vi "Check Alarm-Error Consistency.vi"(8 "error in (no error)":errorcluster, 11 "STEP In":T1) -> (0 "error out":errorcluster, 2 "Array":bool[](array[boolean]), 3 "STEP out":T1)   [LabVIEW 2014, in "SeqLoop.lvlib"]
uses:
  TypeDefs/STEP.ctl
  TypeDefs/LogicParsedExpression.ctl
  Mimico Display/TypeDefs/Mimic Data.ctl
  Mimico Display/TypeDefs/BG Image.ctl
  Mimico Display/TypeDefs/mObject.ctl
  <vilib>/regexp/Match Regular Expression.xnode
  SeqLoop.lvlib
  Mimico Display/Mimico Display.lvlib
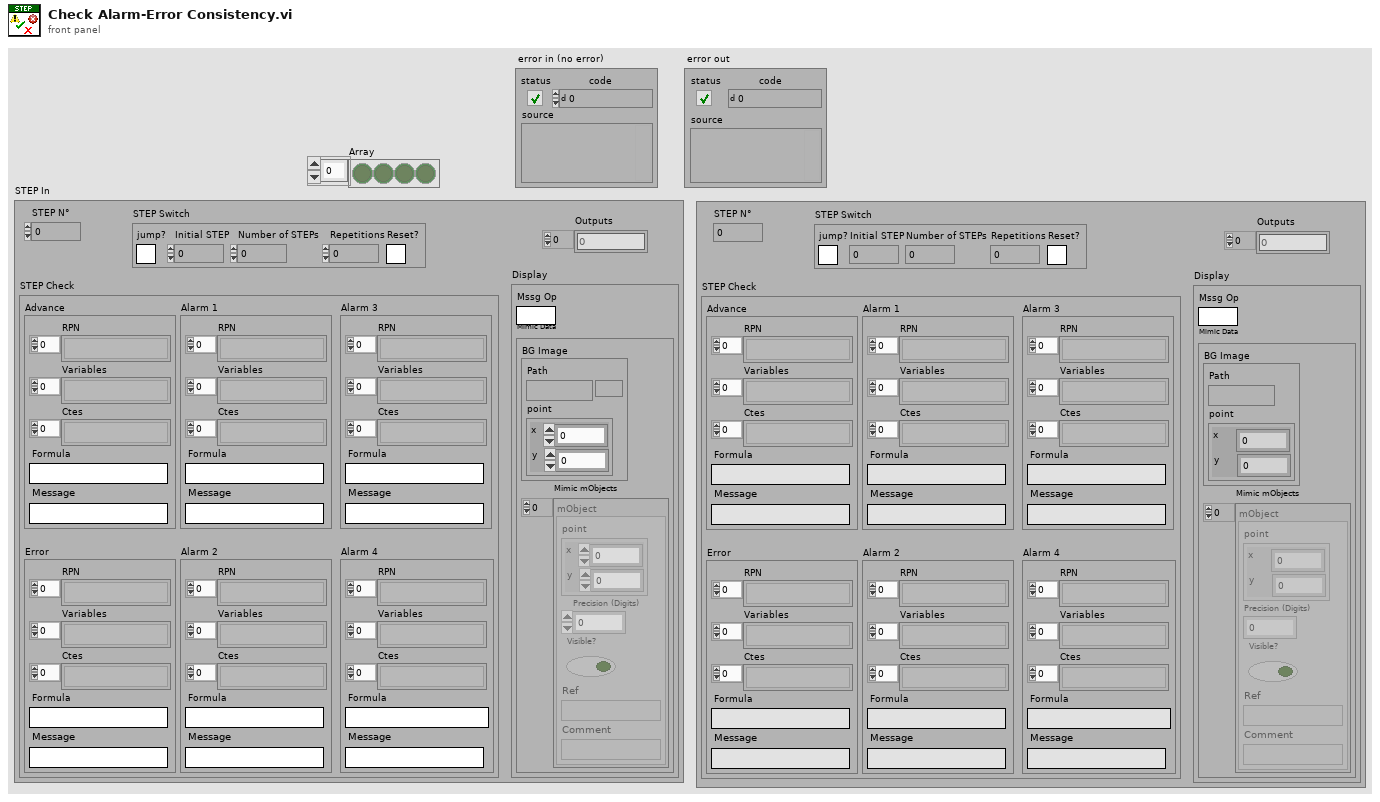
[diagram p1: front panel]
types:
  T1 = typedef "SeqLoop.lvlib/STEP.ctl" = cluster{"STEP N°":u32, "STEP Switch":cluster{"jump?":bool, "Initial STEP":u32, "Number of STEPs":u32, "Repetitions":u32, "Reset?":bool}, "Outputs":i32[], "STEP Check":cluster{"Advance":T2, "Error ":T2, "Alarm 1":T2, "Alarm 2":T2, "Alarm 3":T2, "Alarm 4":T2}, "Display":cluster{"Mssg Op":string, "Mimic Data":T3}}
  T2 = typedef "SeqLoop.lvlib/LogicParsedExpression.ctl" = cluster{"RPN ":string[], "Variables":string[], "Ctes":string[], "Formula":string, "Message":string}
  T3 = typedef "SeqLoop.lvlib/Mimico Display.lvlib/Mimic Data.ctl" = cluster{"BG Image":T4, "Mimic mObjects":T5[]}
  T4 = typedef "SeqLoop.lvlib/Mimico Display.lvlib/BG Image.ctl" = cluster{"Path":path, "point":cluster{"x":i16, "y":i16}}
  T5 = typedef "SeqLoop.lvlib/Mimico Display.lvlib/mObject.ctl" = cluster{"point":cluster{"x":i16, "y":i16}, "Precision (Digits)":i32, "Visible?":bool, "Ref":string, "Comment":string}
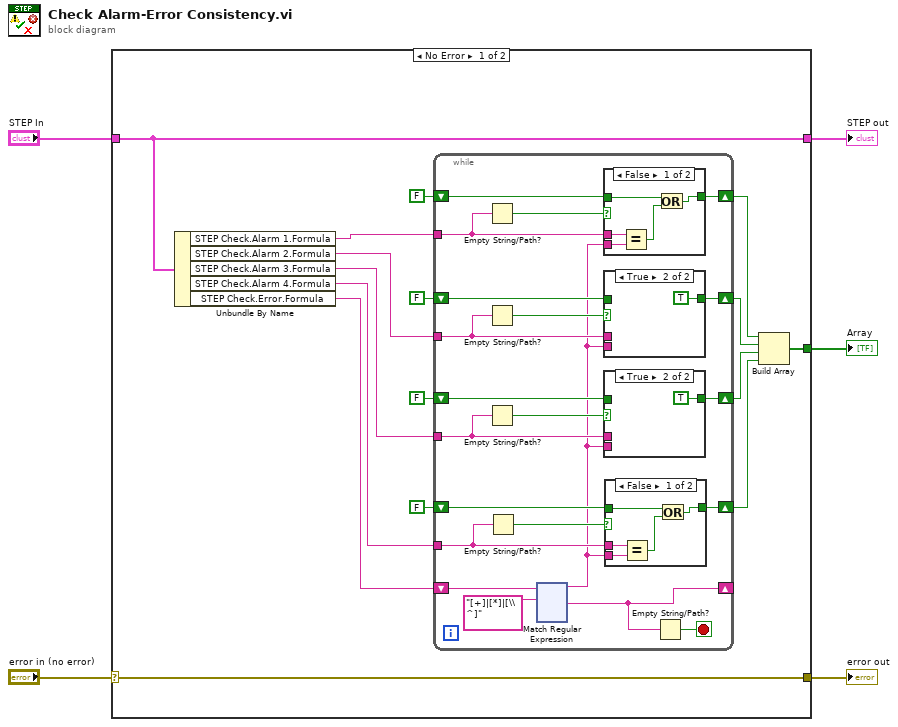
[diagram p0: block diagram]
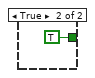
[diagram p2: hidden frame]
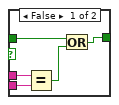
[diagram p3: hidden frame]
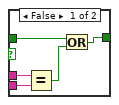
[diagram p4: hidden frame]
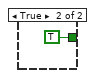
[diagram p5: hidden frame]
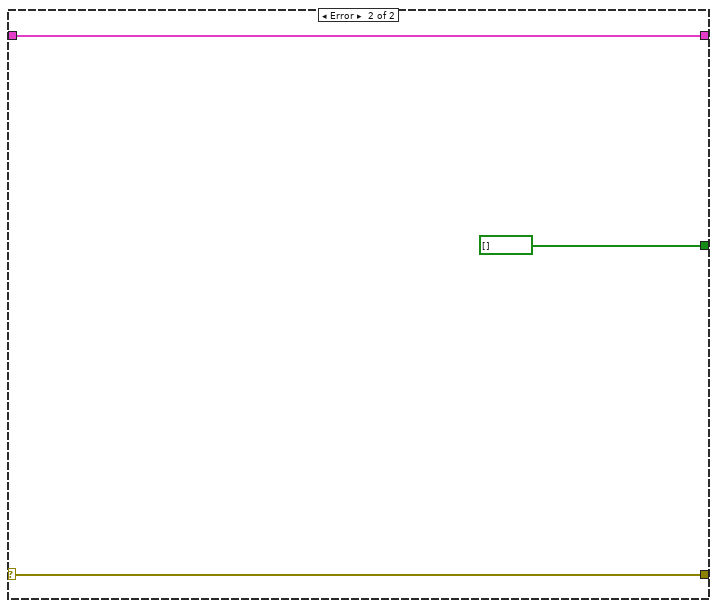
[diagram p6: hidden frame]
diagram:
  n1 = case shown="No Error" "error in (no error)" {
    selector: "error in (no error)" -> [w21 w182]
    tunnel: [w21 w182] -> w4
    tunnel: "STEP In" -> [w11 w183]
    tunnel: [w11 w183] -> w1
    tunnel: [w6 bool[] []] -> w3
    frame No Error {
      n2 = Unbundle By Name(w11) -> ("STEP Check.Alarm 1.Formula"=w16:string, "STEP Check.Alarm 2.Formula"=w17:string, "STEP Check.Alarm 3.Formula"=w18:string, "STEP Check.Alarm 4.Formula"=w19:string, "STEP Check.Error.Formula"=w20:string)
      n3 = while {
        shift-right: [w22] -> _
        shift-left: w20 -> [w24]
        tunnel: w19 -> [w41]
        tunnel: w18 -> [w34]
        tunnel: w17 -> [w33]
        tunnel: w16 -> [w32]
        shift-right: [w40] -> w7
        shift-left: FALSE -> [w39]
        shift-right: [w29] -> w8
        shift-left: FALSE -> [w26]
        shift-right: [w30] -> w9
        shift-left: FALSE -> [w27]
        shift-right: [w31] -> w10
        shift-left: FALSE -> [w28]
        stop <- w38 stop-if-true
        n4 = Empty String/Path?(string/path=w32) -> (empty?=w35:bool)
        n5 = Empty String/Path?(string/path=w33) -> (empty?=w36:bool)
        n6 = Empty String/Path?(string/path=w34) -> (empty?=w37:bool)
        n7 = Empty String/Path?(string/path=w41) -> (empty?=w42:bool)
        n8 = xnode "Match Regular Expression"("input string"=w24, "regular expression"="[+]|[*]|[\\^]") -> ("before match"=w23:string, "after match"=w22:string)  [unwired: 4 in, 3 out]
        n9 = case shown="False" w35 {
          tunnel: w32 -> [w161 _]
          tunnel: w23 -> [w160 _]
          tunnel: w28 -> [w159 _]
          tunnel: [w157 TRUE] -> w31
          frame False {
            n10 = Equal?(x=w161, y=w160) -> (x = y?=w158:bool)
            n11 = Or(x=w159, y=w158) -> (x .or. y?=w157:bool)
          }
          frame True {
          }
        }
        n12 = case shown="True" w36 {
          tunnel: w33 -> [w167 _]
          tunnel: w23 -> [w166 _]
          tunnel: w27 -> [w165 _]
          tunnel: [w163 TRUE] -> w30
          frame False {
            n13 = Equal?(x=w167, y=w166) -> (x = y?=w164:bool)
            n14 = Or(x=w165, y=w164) -> (x .or. y?=w163:bool)
          }
          frame True {
          }
        }
        n15 = case shown="True" w37 {
          tunnel: w34 -> [w173 _]
          tunnel: w23 -> [w172 _]
          tunnel: w26 -> [w171 _]
          tunnel: [w169 TRUE] -> w29
          frame False {
            n16 = Equal?(x=w173, y=w172) -> (x = y?=w170:bool)
            n17 = Or(x=w171, y=w170) -> (x .or. y?=w169:bool)
          }
          frame True {
          }
        }
        n18 = case shown="False" w42 {
          tunnel: w41 -> [w179 _]
          tunnel: w23 -> [w178 _]
          tunnel: w39 -> [w177 _]
          tunnel: [w175 TRUE] -> w40
          frame False {
            n19 = Equal?(x=w179, y=w178) -> (x = y?=w176:bool)
            n20 = Or(x=w177, y=w176) -> (x .or. y?=w175:bool)
          }
          frame True {
          }
        }
        n21 = Empty String/Path?(string/path=w22) -> (empty?=w38:bool)
      }
      n22 = Build Array(w10, w9, w8, w7) -> (w6:bool[])
    }
    frame Error {
    }
  }
  "error out" <- w4
  "Array" <- w3
  "STEP out" <- w1
